vi "Is_Elevator_Move.vi"(8 "error in (no error)":errorcluster, 11 "Elevator in":T1) -> (0 "error out":errorcluster, 2 "Elevator out":T1, 3 "Move?":bool)   [LabVIEW 2026]
uses:
  Controls/Door_Status_Enum.ctl
  Controls/Occupy_Status.ctl
  Controls/Floor_Status.ctl
  Controls/Motion_Status_Enum.ctl
  Controls/Car_Calls_Status.ctl
  Controls/Hall_Calls_Status.ctl
  Controls/Elevator_Status.ctl
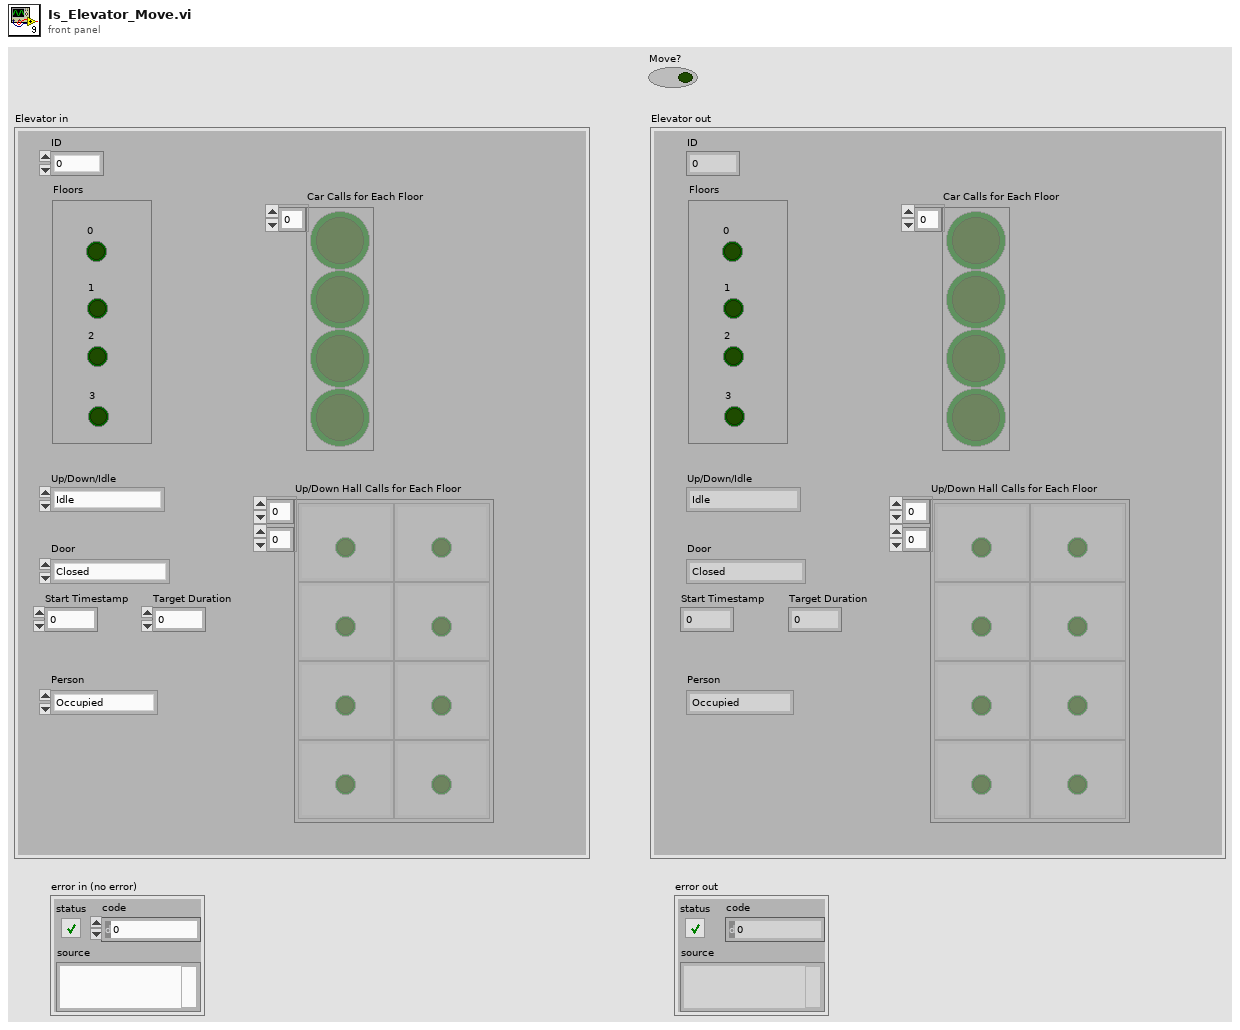
[diagram p1: front panel]
types:
  T1 = typedef "Elevator_Status.ctl" = cluster{"Door":T2, "Person":T3, "Floors":T4, "Up/Down/Idle":T5, "Car Calls for Each Floor":T6, "Up/Down Hall Calls for Each Floor":T7, "ID":i32, "Start Timestamp":u32, "Target Duration":dbl}
  T2 = typedef "Door_Status_Enum.ctl" = enum16{"Closed", "Open", "Opening", "Closing"}
  T3 = typedef "Occupy_Status.ctl" = enum16{"Occupied", "Empty"}
  T4 = typedef "Floor_Status.ctl" = cluster{"0":bool, "1":bool, "2":bool, "3":bool}
  T5 = typedef "Motion_Status_Enum.ctl" = enum16{"Idle", "Up", "Down"}
  T6 = typedef "Car_Calls_Status.ctl" = bool[]
  T7 = typedef "Hall_Calls_Status.ctl" = cluster{bool}[][]
  T8 = enum16{"Check for Any Floor - Car Call", "Check for Specific Floor - Car Call", "Check for Any Floor - Hall Call", "Check for Specific Floor - Hall Call"}
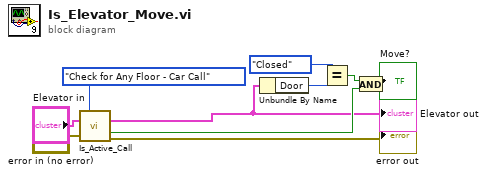
[diagram p0: block diagram]
diagram:
  n1 = call "Is_Active_Call.vi"("Enum"=T8."Check for Any Floor - Car Call", "Elevator in"="Elevator in", "error in (no error)"="error in (no error)") -> ("Elevator out"=w5:T1, "Active Call?"=w9:bool, "error out"=→"error out":errorcluster)  [unwired: 8 in, 2 out]
  "Elevator out" <- w5
  n2 = Unbundle By Name(w5) -> ("Door"=w6:T2)
  n3 = Equal?(x=Door_Status_Enum."Closed", y=w6) -> (x = y?=w8:bool)
  n4 = And(x=w8, y=w9) -> (x .and. y?=→"Move?":bool)
